vi "Max Allowed PDP Currents.vi"() -> ()   [LabVIEW 2017]
panel:
  out "Max Allowed Current":dbl[](array[numeric])
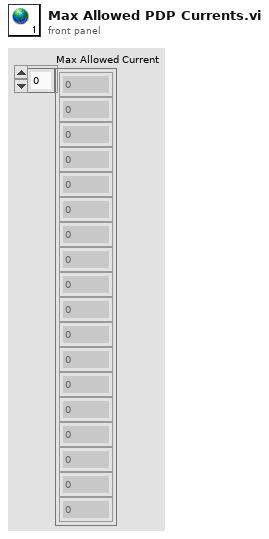
[diagram p1: front panel]
diagram:
